vi "log analysis_gps.vi"() -> ()   [LabVIEW 2019] (continued)
\t269.436139\t81.532625\t9.289600\t-0.460581\t-2.044566\t150.612884\t0.332000\t-0.041000\n\t\n15:34:24.6\tlog_raw\tgps_raw\t\tsystem status\tnormal 2 28.000000 0 0\trobot status\t269.315203\t81.615343\t9.281900\t-0.552229\t-2.021285\t150.644029\t0.244000\t0.082000\n\t\n15:34:25.1\tlog_raw\tgps_raw\t\tsystem status\tnormal 2 28.000000 0 0\trobot status\t269.194622\t81.698654\t9.276300\t-0.583893\t-2.101000\t150.710365\t0.325000\t-0.036000\n\t\n15:34:25.6\tlog_raw\tgps_raw\t\tsystem status\tnormal 2 28.000000 0 0\trobot status\t269.074335\t81.783902\t9.271000\t-0.497675\t-2.181605\t150.744108\t0.241000\t0.088000\n\t\n15:34:26.1\tlog_raw\tgps_raw\t\tsystem status\tnormal 2 28.000000 0 0\trobot status\t268.955477\t81.869341\t9.264900\t-0.452583\t-2.247608\t150.742374\t0.270000\t0.036000\n\t\n15:34:26.6\tlog_raw\tgps_raw\t\tsystem status\tnormal 2 28.000000 0 0\trobot status\t268.833115\t81.953814\t9.258000\t-0.503111\t-2.453600\t150.732052\t0.302000\t-0.013000\n\t\n15:34:27.1\tlog_raw\tgps_raw\t\tsystem status\tnormal 2 28.000000 0 0\trobot status\t268.713878\t82.036962\t9.250800\t-0.577483\t-2.510757\t150.712169\t0.246000\t0.079000\n\t\n15:34:27.6\tlog_raw\tgps_raw\t#INSPVAXA,USB3,0,47.0,FINESTEERING,2107,282885.600,02008000,471d,15824;INS_ALIGNMENT_COMPLETE,INS_RTKFIXED,37.37087024505,126.72386724376,9.2438,22.3000,0.1935,-0.2367,-0.0200,-0.555619573,-2.649892401,299.303581082,0.4421,0.2945,0.5549,0.1137,0.0925,0.0774,0.0981,0.1030,4.8706,0f000001,0*97a1aad7\n\tsystem status\tnormal 2 28.000000 0 0\trobot status\t268.581876\t82.129677\t9.243800\t-0.555620\t-2.649892\t150.696419\t0.296000\t0.008000\n\t\n15:34:28.1\tlog_raw\tgps_raw\t\tsystem status\tnormal 2 28.000000 0 0\trobot status\t268.476510\t82.206619\t9.237300\t-0.368024\t-2.541357\t150.675329\t0.256000\t0.056000\n\t\n15:34:28.6\tlog_raw\tgps_raw\t\tsystem status\tnormal 2 28.000000 0 0\trobot status\t268.358117\t82.289532\t9.231700\t-0.318834\t-2.532121\t150.690435\t0.300000\t0.005000\n\t\n15:34:29.1\tlog_raw\tgps_raw\t\tsystem status\tnormal 2 28.000000 0 0\trobot status\t268.240486\t82.371274\t9.225600\t-0.444676\t-2.457903\t150.683698\t0.361000\t-0.089000\n\t\n15:34:29.6\tlog_raw\tgps_raw\t\tsystem status\tnormal 2 28.000000 0 0\trobot status\t268.120488\t82.453127\t9.219200\t-0.577303\t-2.448788\t150.642594\t0.252000\t0.059000\n\t\n15:34:30.1\tlog_raw\tgps_raw\t#INSPVAXA,USB3,0,44.0,FINESTEERING,2107,282888.100,02000000,471d,15824;INS_ALIGNMENT_COMPLETE,INS_RTKFIXED,37.37087398802,126.72386055207,9.2130,22.3000,0.1784,-0.2231,-0.0172,-0.474670007,-2.406033288,299.373176614,0.4412,0.2944,0.5546,0.1136,0.0925,0.0773,0.0980,0.1030,4.8749,0f000001,0*64b8e8ef\n\tsystem status\tnormal 2 28.000000 0 0\trobot status\t267.989137\t82.545108\t9.213000\t-0.474670\t-2.406033\t150.626823\t0.268000\t0.034000\n\t\n15:34:30.6\tlog_raw\tgps_raw\t\tsystem status\tnormal 2 28.000000 0 0\trobot status\t267.880467\t82.621276\t9.207200\t-0.438602\t-2.378533\t150.618241\t0.244000\t0.081000\n\t\n15:34:31.1\tlog_raw\tgps_raw\t\tsystem status\tnormal 2 28.000000 0 0\trobot status\t267.761451\t82.706078\t9.200700\t-0.346891\t-2.412332\t150.574151\t0.282000\t0.019000\n\t\n15:34:31.6\tlog_raw\tgps_raw\t\tsystem status\tnormal 2 28.000000 0 0\trobot status\t267.643575\t82.787980\t9.195000\t-0.379001\t-2.289734\t150.506519\t0.353000\t-0.088000\n\t\n15:34:32.1\tlog_raw\tgps_raw\t\tsystem status\tnormal 2 28.000000 0 0\trobot status\t267.524465\t82.871251\t9.188700\t-0.470678\t-2.248727\t150.509531\t0.253000\t0.060000\n\t\n15:34:32.6\tlog_raw\tgps_raw\t\tsystem status\tnormal 2 28.000000 0 0\trobot status\t267.407071\t82.952609\t9.183600\t-0.561567\t-2.263237\t150.489005\t0.287000\t0.025000\n\t\n15:34:33.1\tlog_raw\tgps_raw\t\tsystem status\tnormal 2 28.000000 0 0\trobot status\t267.291089\t83.035299\t9.177300\t-0.538205\t-2.174307\t150.443336\t0.289000\t0.018000\n\t\n15:34:33.6\tlog_raw\tgps_raw\t\tsystem status\tnormal 2 28.000000 0 0\trobot status\t267.174248\t83.118918\t9.171300\t-0.308620\t-2.273326\t150.485622\t0.327000\t-0.053000\n\t\n15:34:34.1\tlog_raw\tgps_raw\t\tsystem status\tnormal 2 28.000000 0 0\trobot status\t267.055065\t83.203999\t9.166400\t-0.214815\t-2.374419\t150.446306\t0.363000\t-0.110000\n\t\n15:34:34.6\tlog_raw\tgps_raw\t\tsystem status\tnormal 2 28.000000 0 0\trobot status\t266.938684\t83.285845\t9.161300\t-0.295524\t-2.437327\t150.392182\t0.278000\t0.033000\n\t\n15:34:35.1\tlog_raw\tgps_raw\t\tsystem status\tnormal 2 28.000000 0 0\trobot status\t266.824358\t83.368135\t9.157000\t-0.276386\t-2.328868\t150.443706\t0.279000\t0.029000\n\t\n15:34:35.6\tlog_raw\tgps_raw\t\tsystem status\tnormal 2 28.000000 0 0\trobot status\t266.706166\t83.452437\t9.153400\t-0.267022\t-2.347712\t150.469778\t0.323000\t-0.044000\n\t\n15:34:36.1\tlog_raw\tgps_raw\t\tsystem status\tnormal 2 28.000000 0 0\trobot status\t266.589120\t83.537244\t9.150100\t-0.269755\t-2.340895\t150.478741\t0.285000\t0.026000\n\t\n15:34:36.6\tlog_raw\tgps_raw\t\tsystem status\tnormal 2 28.000000 0 0\trobot status\t266.475594\t83.619238\t9.146900\t-0.192257\t-2.213213\t150.498544\t0.384000\t-0.112000\n\t\n15:34:37.1\tlog_raw\tgps_raw\t#INSPVAXA,USB3,0,48.5,FINESTEERING,2107,282895.100,02000000,471d,15824;INS_ALIGNMENT_COMPLETE,INS_RTKFIXED,37.37088448799,126.72384205034,9.1438,22.3000,0.1933,-0.2424,-0.0028,-0.201390353,-2.093342605,299.449772344,0.4447,0.2945,0.5555,0.1140,0.0925,0.0774,0.0980,0.1030,4.8838,0f000001,0*927e2c09\n\tsystem status\tnormal 2 27.900000 0 0\trobot status\t266.350284\t83.710495\t9.143800\t-0.201390\t-2.093343\t150.550228\t0.262000\t0.069000\n\t\n15:34:37.6\tlog_raw\tgps_raw\t#INSPVAXA,USB3,0,48.5,FINESTEERING,2107,282895.600,02000000,471d,15824;INS_ALIGNMENT_COMPLETE,INS_RTKFIXED,37.37088525085,126.72384071933,9.1382,22.3000,0.1891,-0.2249,-0.0147,-0.298436977,-2.149365506,299.431607145,0.4447,0.2945,0.5555,0.1140,0.0925,0.0774,0.0980,0.1030,4.8838,0f000001,0*8cb89ae5\n\tsystem status\tnormal 2 27.900000 0 0\trobot status\t266.232386\t83.795165\t9.138200\t-0.298437\t-2.149366\t150.568393\t0.281000\t0.032000\n\t\n15:34:38.1\tlog_raw\tgps_raw\t#INSPVAXA,USB3,0,50.0,FINESTEERING,2107,282896.100,02000000,471d,15824;INS_ALIGNMENT_COMPLETE,INS_RTKFIXED,37.37088602098,126.72383942643,9.1321,22.3000,0.1872,-0.2208,-0.0098,-0.216671820,-2.100330729,299.377504290,0.4449,0.2945,0.5555,0.1140,0.0925,0.0774,0.0980,0.1030,4.8845,0f000001,0*ef0b4927\n\tsystem status\tnormal 2 28.000000 0 0\trobot status\t266.117863\t83.880641\t9.132100\t-0.216672\t-2.100331\t150.622496\t0.265000\t0.063000\n\t\n15:34:38.6\tlog_raw\tgps_raw\t#INSPVAXA,USB3,0,50.0,FINESTEERING,2107,282896.600,02000000,471d,15824;INS_ALIGNMENT_COMPLETE,INS_RTKFIXED,37.37088675072,126.72383814980,9.1274,22.3000,0.1877,-0.2084,-0.0156,-0.228208842,-2.023017787,299.331781816,0.4449,0.2945,0.5555,0.1140,0.0925,0.0774,0.0980,0.1030,4.8845,0f000001,0*c594017f\n\tsystem status\tnormal 2 28.000000 0 0\trobot status\t266.004781\t83.961635\t9.127400\t-0.228209\t-2.023018\t150.668218\t0.285000\t0.024000\n\t\n15:34:39.1\tlog_raw\tgps_raw\t#INSPVAXA,USB3,0,50.5,FINESTEERING,2107,282897.100,02000000,471d,15824;INS_ALIGNMENT_COMPLETE,INS_RTKFIXED,37.37088750252,126.72383685308,9.1243,22.3000,0.1876,-0.2107,-0.0114,-0.201079382,-2.183646945,299.196189709,0.4447,0.2943,0.5554,0.1139,0.0925,0.0774,0.0980,0.1030,4.8850,0f000001,0*259ceb0e\n\tsystem status\tnormal 2 28.000000 0 0\trobot status\t265.889920\t84.045076\t9.124300\t-0.201079\t-2.183647\t150.803810\t0.274000\t0.040000\n\t\n15:34:39.6\tlog_raw\tgps_raw\t#INSPVAXA,USB3,0,50.5,FINESTEERING,2107,282897.600,02000000,471d,15824;INS_ALIGNMENT_COMPLETE,INS_RTKFIXED,37.37088825874,126.72383552871,9.1219,22.3000,0.1981,-0.2184,-0.0197,-0.162513691,-2.197478943,299.137776460,0.4447,0.2943,0.5554,0.1139,0.0925,0.0774,0.0980,0.1030,4.8850,0f000001,0*0c5abc39\n\tsystem status\tnormal 2 28.000000 0 0\trobot status\t265.772609\t84.129009\t9.121900\t-0.162514\t-2.197479\t150.862224\t0.353000\t-0.063000\n\t\n15:34:40.1\tlog_raw\tgps_raw\t#INSPVAXA,USB3,0,49.5,FINESTEERING,2107,282898.100,02000000,471d,15824;INS_ALIGNMENT_COMPLETE,INS_RTKFIXED,37.37088900648,126.72383424276,9.1196,22.3000,0.2094,-0.2215,-0.0185,-0.097507181,-2.148657540,298.990101476,0.4444,0.2942,0.5550,0.1138,0.0925,0.0774,0.0981,0.1030,4.8854,0f000001,0*b8bcb2e5\n\tsystem status\tnormal 2 27.900000 0 0\trobot status\t265.658702\t84.212000\t9.119600\t-0.097507\t-2.148658\t151.009899\t0.277000\t0.042000\n\t\n15:34:40.6\tlog_raw\tgps_raw\t\tsystem status\tnormal 2 27.900000 0 0\trobot status\t265.555116\t84.286064\t9.116100\t-0.033377\t-2.065894\t151.068145\t0.247000\t0.094000\n\t\n15:34:41.1\tlog_raw\tgps_raw\t\tsystem status\tnormal 2 28.000000 0 0\trobot status\t265.437719\t84.369636\t9.111700\t-0.021479\t-2.037968\t151.178463\t0.448000\t-0.221000\n\t\n15:34:41.6\tlog_raw\tgps_raw\t\tsystem status\tnormal 2 27.900000 0 0\trobot status\t265.321293\t84.451017\t9.109300\t0.038913\t-2.028452\t151.267255\t0.273000\t0.055000\n\t\n15:34:42.1\tlog_raw\tgps_raw\t\tsystem status\tnormal 2 27.900000 0 0\trobot status\t265.205758\t84.531606\t9.106900\t-0.067838\t-1.982593\t151.367214\t0.234000\t0.111000\n\t\n15:34:42.6\tlog_raw\tgps_raw\t\tsystem status\tnormal 2 27.900000 0 0\trobot status\t265.087725\t84.613924\t9.104700\t0.030629\t-2.066884\t151.494607\t0.249000\t0.072000\n\t\n15:34:43.1\tlog_raw\tgps_raw\t#INSPVAXA,USB3,0,44.5,FINESTEERING,2107,282901.100,02000000,471d,15824;INS_ALIGNMENT_COMPLETE,INS_RTKFIXED,37.37089345276,126.72382632257,9.1013,22.3000,0.2073,-0.2174,-0.0049,0.127947696,-2.049748095,298.428012229,0.4429,0.2942,0.5542,0.1136,0.0924,0.0773,0.0981,0.1029,4.8869,0f000001,0*2739f994\n\tsystem status\tnormal 2 27.900000 0 0\trobot status\t264.957144\t84.705491\t9.101300\t0.127948\t-2.049748\t151.571988\t0.351000\t-0.065000\n\t\n15:34:43.6\tlog_raw\tgps_raw\t#INSPVAXA,USB3,0,44.5,FINESTEERING,2107,282901.600,02000000,471d,15824;INS_ALIGNMENT_COMPLETE,INS_RTKFIXED,37.37089417130,126.72382498099,9.0979,22.3000,0.2123,-0.2139,-0.0112,0.110382768,-2.113702114,298.389030042,0.4429,0.2942,0.5542,0.1136,0.0924,0.0773,0.0981,0.1029,4.8869,0f000001,0*7ea02078\n\tsystem status\tnormal 2 27.900000 0 0\trobot status\t264.838309\t84.785242\t9.097900\t0.110383\t-2.113702\t151.610970\t0.439000\t-0.195000\n\t\n15:34:44.1\tlog_raw\tgps_raw\t#INSPVAXA,USB3,0,47.5,FINESTEERING,2107,282902.100,02000000,471d,15824;INS_ALIGNMENT_COMPLETE,INS_RTKFIXED,37.37089489898,126.72382363217,9.0942,22.3000,0.2058,-0.2206,-0.0113,0.048071178,-2.299077036,298.376589904,0.4428,0.2943,0.5540,0.1136,0.0924,0.0773,0.0981,0.1029,4.8877,0f000001,0*27878755\n\tsystem status\tnormal 2 28.000000 0 0\trobot status\t264.718833\t84.866007\t9.094200\t0.048071\t-2.299077\t151.623410\t0.221000\t0.136000\n\t\n15:34:44.6\tlog_raw\tgps_raw\t#INSPVAXA,USB3,0,47.5,FINESTEERING,2107,282902.600,02000000,471d,15824;INS_ALIGNMENT_COMPLETE,INS_RTKFIXED,37.37089561933,126.72382228336,9.0897,22.3000,0.2051,-0.2120,-0.0118,0.043026481,-2.382631281,298.375025440,0.4428,0.2943,0.5540,0.1136,0.0924,0.0773,0.0981,0.1029,4.8877,0f000001,0*7b155814\n\tsystem status\tnormal 2 28.000000 0 0\trobot status\t264.599358\t84.945958\t9.089700\t0.043026\t-2.382631\t151.624975\t0.344000\t-0.069000\n\t\n15:34:45.1\tlog_raw\tgps_raw\t#INSPVAXA,USB3,0,50.5,FINESTEERING,2107,282903.100,02000000,471d,15824;INS_ALIGNMENT_COMPLETE,INS_RTKFIXED,37.37089633791,126.72382096695,9.0851,22.3000,0.2033,-0.2166,-0.0158,0.077766570,-2.447937912,298.353889057,0.4425,0.2944,0.5540,0.1136,0.0924,0.0773,0.0981,0.1029,4.8888,0f000001,0*d3856956\n\tsystem status\tnormal 2 28.000000 0 0\trobot status\t264.482752\t85.025713\t9.085100\t0.077767\t-2.447938\t151.646111\t0.409000\t-0.173000\n\t\n15:34:45.6\tlog_raw\tgps_raw\t#INSPVAXA,USB3,0,50.5,FINESTEERING,2107,282903.600,02000000,471d,15824;INS_ALIGNMENT_COMPLETE,INS_RTKFIXED,37.37089705589,126.72381965369,9.0797,22.3000,0.2030,-0.2155,-0.0169,0.162662561,-2.490332346,298.323964728,0.4425,0.2944,0.5540,0.1136,0.0924,0.0773,0.0981,0.1029,4.8888,0f000001,0*903bf558\n\tsystem status\tnormal 2 28.000000 0 0\trobot status\t264.366426\t85.105402\t9.079700\t0.162663\t-2.490332\t151.676035\t0.328000\t-0.052000\n\t\n15:34:46.1\tlog_raw\tgps_raw\t#INSPVAXA,USB3,0,48.5,FINESTEERING,2107,282904.100,02000000,471d,15824;INS_ALIGNMENT_COMPLETE,INS_RTKFIXED,37.37089779647,126.72381832272,9.0739,22.3000,0.1899,-0.2136,-0.0154,0.294805164,-2.652846307,298.299564354,0.4429,0.2945,0.5544,0.1137,0.0925,0.0774,0.0981,0.1030,4.8900,0f000001,0*1aba8cff\n\tsystem status\tnormal 2 28.000000 0 0\trobot status\t264.248531\t85.187598\t9.073900\t0.294805\t-2.652846\t151.700436\t0.281000\t0.007000\n\t\n15:34:46.6\tlog_raw\tgps_raw\t\tsystem status\tnormal 2 28.000000 0 0\trobot status\t264.139827\t85.260598\t9.068300\t0.313257\t-2.570583\t151.646867\t0.257000\t0.059000\n\t\n15:34:47.1\tlog_raw\tgps_raw\t#INSPVAXA,USB3,0,42.5,FINESTEERING,2107,282905.100,02000000,471d,15824;INS_ALIGNMENT_COMPLETE,INS_RTKFIXED,37.37089924281,126.72381565825,9.0621,22.3000,0.2032,-0.2264,-0.0151,0.296199790,-2.500120429,298.405278935,0.4415,0.2943,0.5538,0.1135,0.0924,0.0773,0.0981,0.1029,4.8913,0f000001,0*c27d96a4\n\tsystem status\tnormal 2 28.000000 0 0\trobot status\t264.012516\t85.348127\t9.062100\t0.296200\t-2.500120\t151.594721\t0.253000\t0.070000\n\t\n15:34:47.6\tlog_raw\tgps_raw\t#INSPVAXA,USB3,0,42.5,FINESTEERING,2107,282905.600,02000000,471d,15824;INS_ALIGNMENT_COMPLETE,INS_RTKFIXED,37.37089993990,126.72381433650,9.0561,22.3000,0.1965,-0.2206,-0.0194,0.175024687,-2.429152117,298.413626254,0.4415,0.2943,0.5538,0.1135,0.0924,0.0773,0.0981,0.1029,4.8913,0f000001,0*60204f40\n\tsystem status\tnormal 2 28.000000 0 0\trobot status\t263.895438\t85.425497\t9.056100\t0.175025\t-2.429152\t151.586374\t0.255000\t0.060000\n\t\n15:34:48.1\tlog_raw\tgps_raw\t#INSPVAXA,USB3,0,50.0,FINESTEERING,2107,282906.100,02000000,471d,15824;INS_ALIGNMENT_COMPLETE,INS_RTKFIXED,37.37090067392,126.72381297631,9.0488,22.3000,0.1869,-0.2231,-0.0278,0.198226586,-2.470510374,298.476445158,0.4408,0.2943,0.5536,0.1134,0.0924,0.0773,0.0981,0.1029,4.8926,0f000001,0*c8d31ab7\n\tsystem status\tnormal 2 28.000000 0 0\trobot status\t263.774954\t85.506966\t9.048800\t0.198227\t-2.470510\t151.523555\t0.243000\t0.074000\n\t\n15:34:48.6\tlog_raw\tgps_raw\t#INSPVAXA,USB3,0,50.0,FINESTEERING,2107,282906.600,02000000,471d,15824;INS_ALIGNMENT_COMPLETE,INS_RTKFIXED,37.37090140156,126.72381162044,9.0410,22.3000,0.1900,-0.2268,-0.0250,0.233406583,-2.464396388,298.527307451,0.4408,0.2943,0.5536,0.1134,0.0924,0.0773,0.0981,0.1029,4.8926,0f000001,0*6dbb954e\n\tsystem status\tnormal 2 28.000000 0 0\trobot status\t263.654854\t85.587727\t9.041000\t0.233407\t-2.464396\t151.472693\t0.249000\t0.074000\n\t\n15:34:49.1\tlog_raw\tgps_raw\t#INSPVAXA,USB3,0,47.5,FINESTEERING,2107,282907.100,02000000,471d,15824;INS_ALIGNMENT_COMPLETE,INS_RTKFIXED,37.37090211288,126.72381031698,9.0345,22.3000,0.1914,-0.2193,-0.0163,0.234265658,-2.429917565,298.557656131,0.4407,0.2944,0.5534,0.1135,0.0925,0.0773,0.0981,0.1029,4.8940,0f000001,0*98d66c71\n\tsystem status\tnormal 2 28.000000 0 0\trobot status\t263.539395\t85.666676\t9.034500\t0.234266\t-2.429918\t151.442344\t0.281000\t0.006000\n\t\n15:34:49.6\tlog_raw\tgps_raw\t#INSPVAXA,USB3,0,47.5,FINESTEERING,2107,282907.600,02000000,471d,15824;INS_ALIGNMENT_COMPLETE,INS_RTKFIXED,37.37090284953,126.72380892748,9.0281,22.3000,0.1780,-0.2041,-0.0150,0.112459051,-2.561733911,298.657756217,0.4407,0.2944,0.5534,0.1135,0.0925,0.0773,0.0981,0.1029,4.8940,0f000001,0*46e93b24\n\tsystem status\tnormal 2 28.000000 0 0\trobot status\t263.416316\t85.748437\t9.028100\t0.112459\t-2.561734\t151.342244\t0.249000\t0.069000\n\t\n15:34:50.1\tlog_raw\tgps_raw\t#INSPVAXA,USB3,0,47.5,FINESTEERING,2107,282908.100,02000000,471d,15824;INS_ALIGNMENT_COMPLETE,INS_RTKFIXED,37.37090357557,126.72380757332,9.0217,22.3000,0.2057,-0.2321,-0.0149,0.061524953,-2.489801509,298.773706778,0.4409,0.2944,0.5534,0.1134,0.0925,0.0773,0.0981,0.1029,4.8951,0f000001,0*737dd3e1\n\tsystem status\tnormal 2 28.000000 0 0\trobot status\t263.296366\t85.829020\t9.021700\t0.061525\t-2.489802\t151.226293\t0.296000\t0.003000\n\t\n15:34:50.6\tlog_raw\tgps_raw\t#INSPVAXA,USB3,0,42.5,FINESTEERING,2107,282908.600,02000000,471d,15824;INS_ALIGNMENT_COMPLETE,INS_RTKFIXED,37.37090428415,126.72380622581,9.0150,22.3000,0.1993,-0.2229,-0.0194,0.018544103,-2.459857959,298.845685977,0.4409,0.2944,0.5534,0.1134,0.0925,0.0773,0.0981,0.1029,4.8951,0f000001,0*f932705e\n\tsystem status\tnormal 2 28.000000 0 0\trobot status\t263.177006\t85.907665\t9.015000\t0.018544\t-2.459858\t151.154314\t0.276000\t0.024000\n\t\n15:34:51.1\tlog_raw\tgps_raw\t#INSPVAXA,USB3,0,45.5,FINESTEERING,2107,282909.100,02000000,471d,15824;INS_ALIGNMENT_COMPLETE,INS_RTKFIXED,37.37090502254,126.72380483216,9.0074,22.3000,0.1877,-0.2104,-0.0206,-0.090329657,-2.475798603,298.940458629,0.4409,0.2946,0.5535,0.1135,0.0926,0.0773,0.0981,0.1029,4.8962,0f000001,0*a1f88c2d\n\tsystem status\tnormal 2 28.000000 0 0\trobot status\t263.053559\t85.989619\t9.007400\t-0.090330\t-2.475799\t151.059541\t0.249000\t0.062000\n\t\n15:34:51.6\tlog_raw\tgps_raw\t#INSPVAXA,USB3,0,45.5,FINESTEERING,2107,282909.600,02000000,471d,15824;INS_ALIGNMENT_COMPLETE,INS_RTKFIXED,37.37090578020,126.72380341402,9.0005,22.3000,0.2042,-0.2452,-0.0267,-0.096054371,-2.657817318,299.053399996,0.4409,0.2946,0.5535,0.1135,0.0926,0.0773,0.0981,0.1029,4.8962,0f000001,0*97d4220e\n\tsystem status\tnormal 2 28.000000 0 0\trobot status\t262.927942\t86.073711\t9.000500\t-0.096054\t-2.657817\t150.946600\t0.311000\t-0.024000\n\t\n15:34:52.1\tlog_raw\tgps_raw\t#INSPVAXA,USB3,0,44.5,FINESTEERING,2107,282910.100,02000000,471d,15824;INS_ALIGNMENT_COMPLETE,INS_RTKFIXED,37.37090649384,126.72380213526,8.9945,22.3000,0.1796,-0.2032,-0.0123,-0.081156055,-2.596786574,299.082136119,0.4412,0.2947,0.5535,0.1135,0.0926,0.0773,0.0981,0.1029,4.8970,0f000001,0*70e9c9df\n\tsystem status\tnormal 2 28.000000 0 0\trobot status\t262.814672\t86.152918\t8.994500\t-0.081156\t-2.596787\t150.917864\t0.270000\t0.031000\n\t\n15:34:52.6\tlog_raw\tgps_raw\t#INSPVAXA,USB3,0,44.5,FINESTEERING,2107,282910.600,02000000,471d,15824;INS_ALIGNMENT_COMPLETE,INS_RTKFIXED,37.37090728426,126.72380074897,8.9873,22.3000,0.2078,-0.2346,-0.0218,0.045801771,-2.674891598,299.142927174,0.4412,0.2947,0.5535,0.1135,0.0926,0.0773,0.0981,0.1029,4.8970,0f000001,0*500925c1\n\tsystem status\tnormal 2 28.000000 0 0\trobot status\t262.691877\t86.240646\t8.987300\t0.045802\t-2.674892\t150.857073\t0.306000\t-0.009000\n\t\n15:34:53.1\tlog_raw\tgps_raw\t#INSPVAXA,USB3,0,45.5,FINESTEERING,2107,282911.100,02000000,471d,15824;INS_ALIGNMENT_COMPLETE,INS_RTKFIXED,37.37090803309,126.72379945819,8.9800,22.3000,0.1796,-0.1956,-0.0242,0.023894528,-2.705451433,299.250076985,0.4415,0.2948,0.5535,0.1135,0.0925,0.0773,0.0981,0.1029,4.8973,0f000001,0*fcb889be\n\tsystem status\tnormal 2 28.000000 0 0\trobot status\t262.577542\t86.323758\t8.980000\t0.023895\t-2.705451\t150.749923\t0.328000\t-0.060000\n\t\n15:34:53.6\tlog_raw\tgps_raw\t#INSPVAXA,USB3,0,45.5,FINESTEERING,2107,282911.600,02000000,471d,15824;INS_ALIGNMENT_COMPLETE,INS_RTKFIXED,37.37090882517,126.72379803977,8.9729,22.3000,0.1992,-0.2347,-0.0122,-0.052701655,-2.537774269,299.314444801,0.4415,0.2948,0.5535,0.1135,0.0925,0.0773,0.0981,0.1029,4.8973,0f000001,0*f806d9f3\n\tsystem status\tnormal 2 28.000000 0 0\trobot status\t262.451900\t86.411671\t8.972900\t-0.052702\t-2.537774\t150.685555\t0.302000\t-0.007000\n\t\n15:34:54.1\tlog_raw\tgps_raw\t#INSPVAXA,USB3,0,49.0,FINESTEERING,2107,282912.100,02000000,471d,15824;INS_ALIGNMENT_COMPLETE,INS_RTKFIXED,37.37090954144,126.72379680635,8.9662,22.3000,0.2005,-0.2326,-0.0241,-0.125797305,-2.436851943,299.381095140,0.4412,0.2948,0.5534,0.1134,0.0926,0.0773,0.0980,0.1029,4.8978,0f000001,0*e5b9f40a\n\tsystem status\tnormal 2 28.000000 0 0\trobot status\t262.342646\t86.491169\t8.966200\t-0.125797\t-2.436852\t150.618905\t0.288000\t0.006000\n\t\n15:34:54.6\tlog_raw\tgps_raw\t#INSPVAXA,USB3,0,49.0,FINESTEERING,2107,282912.600,02000000,471d,15824;INS_ALIGNMENT_COMPLETE,INS_RTKFIXED,37.37091031837,126.72379541279,8.9597,22.3000,0.1852,-0.2068,-0.0204,-0.071142448,-2.486574172,299.492569727,0.4412,0.2948,0.5534,0.1134,0.0926,0.0773,0.0980,0.1029,4.8978,0f000001,0*cac4ba0d\n\tsystem status\tnormal 2 28.000000 0 0\trobot status\t262.219207\t86.577401\t8.959700\t-0.071142\t-2.486574\t150.507430\t0.229000\t0.086000\n\t\n15:34:55.1\tlog_raw\tgps_raw\t#INSPVAXA,USB3,0,49.5,FINESTEERING,2107,282913.100,02000000,471d,15824;INS_ALIGNMENT_COMPLETE,INS_RTKFIXED,37.37091108524,126.72379405931,8.9519,22.3000,0.1888,-0.2272,-0.0247,-0.028725670,-2.337365397,299.552597059,0.4407,0.2948,0.5532,0.1133,0.0925,0.0773,0.0980,0.1028,4.8983,0f000001,0*e96bcee1\n\tsystem status\tnormal 2 28.000000 0 0\trobot status\t262.099318\t86.662515\t8.951900\t-0.028726\t-2.337365\t150.447403\t0.289000\t0.015000\n\t\n15:34:55.6\tlog_raw\tgps_raw\t#INSPVAXA,USB3,0,49.5,FINESTEERING,2107,282913.600,02000000,471d,15824;INS_ALIGNMENT_COMPLETE,INS_RTKFIXED,37.37091181929,126.72379275953,8.9460,22.3000,0.2010,-0.2341,-0.0266,0.089811982,-2.060196464,299.576677056,0.4407,0.2948,0.5532,0.1133,0.0925,0.0773,0.0980,0.1028,4.8983,0f000001,0*1320fd5f\n\tsystem status\tnormal 2 28.000000 0 0\trobot status\t261.984185\t86.743987\t8.946000\t0.089812\t-2.060196\t150.423323\t0.349000\t-0.076000\n\t\n15:34:56.1\tlog_raw\tgps_raw\t#DUALANTENNAHEADINGA,USB3,0,49.5,FINESTEERING,2107,282914.100,02000000,d426,15824;INSUFFICIENT_OBS,NONE,-1.000000000,0.000000000,0.000000000,0.0,0.000000000,0.000000000,\"631T\",13,2,2,2,04,00,20,00*7d7777a8\n\tsystem status\tnormal 2 28.000000 0 0\trobot status\t261.864200\t86.827130\t8.939200\t-0.070666\t-2.033883\t150.415109\t0.253000\t0.066000\n\t\n15:34:56.6\tlog_raw\tgps_raw\t#INSPVAXA,USB3,0,52.5,FINESTEERING,2107,282914.600,02000000,471d,15824;INS_ALIGNMENT_COMPLETE,INS_RTKFIXED,37.37091330951,126.72379003668,8.9325,22.3000,0.2030,-0.2221,-0.0237,-0.171357010,-2.043364935,299.558430803,0.4402,0.2946,0.5530,0.1134,0.0925,0.0773,0.0980,0.1028,4.8991,0f000001,0*e9175f83\n\tsystem status\tnormal 2 28.000000 0 0\trobot status\t261.743000\t86.909386\t8.932500\t-0.171357\t-2.043365\t150.441569\t0.258000\t0.063000\n\t\n15:34:57.1\tlog_raw\tgps_raw\t#INSPVAXA,USB3,0,50.0,FINESTEERING,2107,282915.100,02000000,471d,15824;INS_ALIGNMENT_COMPLETE,INS_RTKFIXED,37.37091408421,126.72378863973,8.9262,22.3000,0.1969,-0.2337,-0.0140,-0.095383380,-2.265013961,299.603418262,0.4401,0.2946,0.5529,0.1132,0.0924,0.0773,0.0980,0.1028,4.8997,0f000001,0*6f852fd6\n\tsystem status\tnormal 2 28.000000 0 0\trobot status\t261.619260\t86.995370\t8.926200\t-0.095383\t-2.265014\t150.396582\t0.255000\t0.060000\n\t\n15:34:57.6\tlog_raw\tgps_raw\t#DUALANTENNAHEADINGA,USB3,0,50.0,FINESTEERING,2107,282915.600,02000000,d426,15824;INSUFFICIENT_OBS,NONE,-1.000000000,0.000000000,0.000000000,0.0,0.000000000,0.000000000,\"631T\",17,2,2,2,04,00,20,00*414acee8\n\tsystem status\tnormal 2 28.000000 0 0\trobot status\t261.500918\t87.077460\t8.921500\t-0.059833\t-2.292781\t150.397040\t0.297000\t0.006000\n\t\n15:34:58.1\tlog_raw\tgps_raw\t#DUALANTENNAHEADINGA,USB3,0,48.5,FINESTEERING,2107,282916.100,02000000,d426,15824;INSUFFICIENT_OBS,NONE,-1.000000000,0.000000000,0.000000000,0.0,0.000000000,0.000000000,\"631T\",16,2,2,2,04,00,20,00*fc092504\n\tsystem status\tnormal 2 28.000000 0 0\trobot status\t261.379338\t87.160459\t8.916300\t-0.201226\t-2.330521\t150.547227\t0.285000\t0.028000\n\t\n15:34:58.6\tlog_raw\tgps_raw\t#INSPVAXA,USB3,0,48.5,FINESTEERING,2107,282916.600,02000000,471d,15824;INS_ALIGNMENT_COMPLETE,INS_RTKFIXED,37.37091631932,126.72378455605,8.9095,22.3000,0.1948,-0.2448,-0.0204,-0.186363479,-2.427120198,299.446159990,0.4395,0.2945,0.5529,0.1132,0.0924,0.0773,0.0979,0.1028,4.9009,0f000001,0*c1989546\n\tsystem status\tnormal 2 28.000000 0 0\trobot status\t261.257534\t87.243444\t8.909500\t-0.186363\t-2.427120\t150.553840\t0.289000\t0.009000\n\t\n15:34:59.1\tlog_raw\tgps_raw\t#INSPVAXA,USB3,0,49.0,FINESTEERING,2107,282917.100,02000000,471d,15824;INS_ALIGNMENT_COMPLETE,INS_RTKFIXED,37.37091707280,126.72378318034,8.9014,22.3000,0.1962,-0.2403,-0.0192,-0.090528151,-2.520576171,299.333268916,0.4392,0.2943,0.5527,0.1132,0.0925,0.0773,0.0979,0.1028,4.9023,0f000001,0*ed058076\n\tsystem status\tnormal 2 27.900000 0 0\trobot status\t261.135676\t87.327072\t8.901400\t-0.090528\t-2.520576\t150.666731\t0.298000\t-0.006000\n\t\n15:34:59.6\tlog_raw\tgps_raw\t#INSPVAXA,USB3,0,49.0,FINESTEERING,2107,282917.600,02000000,471d,15824;INS_ALIGNMENT_COMPLETE,INS_RTKFIXED,37.37091780195,126.72378182721,8.8930,22.3000,0.1904,-0.2448,-0.0126,-0.105477255,-2.530837408,299.214922397,0.4392,0.2943,0.5527,0.1132,0.0925,0.0773,0.0979,0.1028,4.9023,0f000001,0*48e5530c\n\tsystem status\tnormal 2 28.000000 0 0\trobot status\t261.015818\t87.408000\t8.893000\t-0.105477\t-2.530837\t150.785078\t0.219000\t0.123000\n\t\n15:35:00.1\tlog_raw\tgps_raw\t#INSPVAXA,USB3,0,49.5,FINESTEERING,2107,282918.100,02000000,471d,15824;INS_ALIGNMENT_COMPLETE,INS_RTKFIXED,37.37091853728,126.72378045121,8.8866,22.3000,0.1905,-0.2390,-0.0217,-0.320620124,-2.745936216,299.166142272,0.4393,0.2944,0.5528,0.1133,0.0925,0.0773,0.0979,0.1028,4.9038,0f000001,0*f3e51291\n\tsystem status\tnormal 2 28.000000 0 0\trobot status\t260.893934\t87.489614\t8.886600\t-0.320620\t-2.745936\t150.833858\t0.298000\t0.003000\n\t\n15:35:00.6\tlog_raw\tgps_raw\t#INSPVAXA,USB3,0,49.5,FINESTEERING,2107,282918.600,02000000,471d,15824;INS_ALIGNMENT_COMPLETE,INS_RTKFIXED,37.37091927039,126.72377907949,8.8817,22.3000,0.1978,-0.2407,-0.0282,-0.339255571,-2.778752767,299.132032456,0.4393,0.2944,0.5528,0.1133,0.0925,0.0773,0.0979,0.1028,4.9038,0f000001,0*ae621dff\n\tsystem status\tnormal 2 28.000000 0 0\trobot status\t260.772430\t87.570982\t8.881700\t-0.339256\t-2.778753\t150.867968\t0.431000\t-0.195000\n\t\n15:35:01.1\tlog_raw\tgps_raw\t#INSPVAXA,USB3,0,45.0,FINESTEERING,2107,282919.100,02000000,471d,15824;INS_ALIGNMENT_COMPLETE,INS_RTKFIXED,37.37092001431,126.72377771681,8.8758,22.3000,0.1914,-0.2350,-0.0323,-0.346867597,-2.754638155,299.109102683,0.4397,0.2944,0.5532,0.1134,0.0925,0.0773,0.0979,0.1029,4.9053,0f000001,0*63db1984\n\tsystem status\tnormal 2 27.900000 0 0\trobot status\t260.651726\t87.653550\t8.875800\t-0.346868\t-2.754638\t150.890897\t0.350000\t-0.072000\n\t\n15:35:01.6\tlog_raw\tgps_raw\t#INSPVAXA,USB3,0,45.0,FINESTEERING,2107,282919.600,02000000,471d,15824;INS_ALIGNMENT_COMPLETE,INS_RTKFIXED,37.37092075682,126.72377638763,8.8692,22.3000,0.1933,-0.2372,-0.0282,-0.392529438,-2.688019024,299.098365705,0.4397,0.2944,0.5532,0.1134,0.0925,0.0773,0.0979,0.1029,4.9053,0f000001,0*15ef86f5\n\tsystem status\tnormal 2 28.000000 0 0\trobot status\t260.533989\t87.735960\t8.869200\t-0.392529\t-2.688019\t150.901634\t0.326000\t-0.035000\n\t\n15:35:02.1\tlog_raw\tgps_raw\t#INSPVAXA,USB3,0,45.0,FINESTEERING,2107,282920.100,02000000,471d,15824;INS_ALIGNMENT_COMPLETE,INS_RTKFIXED,37.37092151983,126.72377503879,8.8627,22.3000,0.1947,-0.2324,-0.0288,-0.374754303,-2.758160229,299.096118379,0.4395,0.2945,0.5534,0.1133,0.0925,0.0773,0.0980,0.1029,4.9066,0f000001,0*6a5bdc77\n\tsystem status\tnormal 2 28.000000 0 0\trobot status\t260.414511\t87.820647\t8.862700\t-0.374754\t-2.758160\t150.903882\t0.418000\t-0.168000\n\t\n15:35:02.6\tlog_raw\tgps_raw\t#INSPVAXA,USB3,0,50.0,FINESTEERING,2107,282920.600,02000000,471d,15824;INS_ALIGNMENT_COMPLETE,INS_RTKFIXED,37.37092225918,126.72377371320,8.8579,22.3000,0.2080,-0.2433,-0.0263,-0.353123452,-2.702710853,299.168531612,0.4395,0.2945,0.5534,0.1133,0.0925,0.0773,0.0980,0.1029,4.9066,0f000001,0*b7196621\n\tsystem status\tnormal 2 28.000000 0 0\trobot status\t260.297092\t87.902707\t8.857900\t-0.353123\t-2.702711\t150.831468\t0.294000\t0.019000\n\t\n15:35:03.1\tlog_raw\tgps_raw\t#DUALANTENNAHEADINGA,USB3,0,50.0,FINESTEERING,2107,282921.100,02000000,d426,15824;INSUFFICIENT_OBS,NONE,-1.000000000,0.000000000,0.000000000,0.0,0.000000000,0.000000000,\"631T\",10,2,2,2,04,00,20,00*711b9acd\n\tsystem status\tnormal 2 28.000000 0 0\trobot status\t260.180847\t87.984238\t8.853900\t-0.343319\t-2.734939\t150.851400\t0.286000\t0.026000\n\t\n15:35:03.6\tlog_raw\tgps_raw\t#INSPVAXA,USB3,0,51.0,FINESTEERING,2107,282921.600,02000000,471d,15824;INS_ALIGNMENT_COMPLETE,INS_RTKFIXED,37.37092372084,126.72377106985,8.8494,22.3000,0.2060,-0.2301,-0.0270,-0.435271636,-2.731976151,299.129546059,0.4391,0.2944,0.5533,0.1133,0.0925,0.0773,0.0980,0.1029,4.9078,0f000001,0*5c44fd03\n\tsystem status\tnormal 2 28.000000 0 0\trobot status\t260.062949\t88.064936\t8.849400\t-0.435272\t-2.731976\t150.870454\t0.376000\t-0.116000\n\t\n15:35:04.1\tlog_raw\tgps_raw\t#DUALANTENNAHEADINGA,USB3,0,51.0,FINESTEERING,2107,282922.100,02000000,d426,15824;INSUFFICIENT_OBS,NONE,-1.000000000,0.000000000,0.000000000,0.0,0.000000000,0.000000000,\"631T\",12,2,2,2,04,00,20,00*d78347f3\n\tsystem status\tnormal 2 28.000000 0 0\trobot status\t259.944761\t88.147198\t8.844200\t-0.331286\t-2.658657\t150.844836\t0.286000\t0.017000\n\t\n15:35:04.6\tlog_raw\tgps_raw\t#INSPVAXA,USB3,0,51.0,FINESTEERING,2107,282922.600,02000000,471d,15824;INS_ALIGNMENT_COMPLETE,INS_RTKFIXED,37.37092515994,126.72376843182,8.8389,22.3000,0.2111,-0.2302,-0.0297,-0.438503525,-2.449777885,299.109289893,0.4389,0.2944,0.5534,0.1132,0.0925,0.0773,0.0980,0.1029,4.9089,0f000001,0*6200cf77\n\tsystem status\tnormal 2 28.000000 0 0\trobot status\t259.829276\t88.224661\t8.838900\t-0.438504\t-2.449778\t150.890710\t0.250000\t0.077000\n\t\n15:35:05.1\tlog_raw\tgps_raw\t#DUALANTENNAHEADINGA,USB3,0,50.0,FINESTEERING,2107,282923.100,02000000,d426,15824;INSUFFICIENT_OBS,NONE,-1.000000000,0.000000000,0.000000000,0.0,0.000000000,0.000000000,\"631T\",13,2,2,2,04,00,20,00*09fd15d6\n\tsystem status\tnormal 2 28.000000 0 0\trobot status\t259.712506\t88.304900\t8.833600\t-0.400717\t-2.470513\t150.946486\t0.334000\t-0.046000\n\t\n15:35:05.6\tlog_raw\tgps_raw\t#INSPVAXA,USB3,0,50.0,FINESTEERING,2107,282923.600,02000000,471d,15824;INS_ALIGNMENT_COMPLETE,INS_RTKFIXED,37.37092659742,126.72376579558,8.8280,22.3000,0.2079,-0.2335,-0.0340,-0.348522367,-2.471236219,299.076821205,0.4391,0.2944,0.5534,0.1132,0.0924,0.0773,0.0980,0.1029,4.9102,0f000001,0*b1b4b9cc\n\tsystem status\tnormal 2 28.000000 0 0\trobot status\t259.595763\t88.384206\t8.828000\t-0.348522\t-2.471236\t150.923179\t0.335000\t-0.054000\n\t\n15:35:06.1\tlog_raw\tgps_raw\t#DUALANTENNAHEADINGA,USB3,0,50.0,FINESTEERING,2107,282924.100,02000000,d426,15824;INSUFFICIENT_OBS,NONE,-1.000000000,0.000000000,0.000000000,0.0,0.000000000,0.000000000,\"631T\",13,2,2,2,04,00,20,00*d3840d98\n\tsystem status\tnormal 2 28.000000 0 0\trobot status\t259.476998\t88.464105\t8.821800\t-0.401477\t-2.556277\t150.962011\t0.249000\t0.082000\n\t\n15:35:06.6\tlog_raw\tgps_raw\t#DUALANTENNAHEADINGA,USB3,0,51.0,FINESTEERING,2107,282924.600,02000000,d426,15824;INSUFFICIENT_OBS,NONE,-1.000000000,0.000000000,0.000000000,0.0,0.000000000,0.000000000,\"631T\",13,2,2,2,04,00,20,00*7b68c1aa\n\tsystem status\tnormal 2 28.000000 0 0\trobot status\t259.359956\t88.542489\t8.815500\t-0.491575\t-2.591134\t150.972893\t0.250000\t0.082000\n\t\n15:35:07.1\tlog_raw\tgps_raw\t#INSPVAXA,USB3,0,51.5,FINESTEERING,2107,282925.100,02008000,471d,15824;INS_ALIGNMENT_COMPLETE,INS_RTKFIXED,37.37092873619,126.72376179523,8.8090,22.3000,0.2069,-0.2351,-0.0215,-0.632285534,-2.693701140,299.016215129,0.4401,0.2945,0.5538,0.1133,0.0925,0.0773,0.0980,0.1029,4.9131,0f000001,0*70f1efa8\n\tsystem status\tnormal 2 28.000000 0 0\trobot status\t259.241418\t88.621588\t8.809000\t-0.632286\t-2.693701\t150.983785\t0.362000\t-0.083000\n\t\n15:35:07.6\tlog_raw\tgps_raw\t#DUALANTENNAHEADINGA,USB3,0,51.5,FINESTEERING,2107,282925.600,02008000,d426,15824;INSUFFICIENT_OBS,NONE,-1.000000000,0.000000000,0.000000000,0.0,0.000000000,0.000000000,\"631T\",13,2,2,2,04,00,20,00*5559a71e\n\tsystem status\tnormal 2 28.000000 0 0\trobot status\t259.124103\t88.700587\t8.803100\t-0.569231\t-2.829073\t150.996185\t0.311000\t-0.032000\n\t\n15:35:08.1\tlog_raw\tgps_raw\t#DUALANTENNAHEADINGA,USB3,0,49.5,FINESTEERING,2107,282926.100,02008000,d426,15824;INSUFFICIENT_OBS,NONE,-1.000000000,0.000000000,0.000000000,0.0,0.000000000,0.000000000,\"631T\",14,2,2,2,04,00,20,00*20bca12d\n\tsystem status\tnormal 2 28.000000 0 0\trobot status\t259.006675\t88.779598\t8.797200\t-0.565146\t-2.883992\t150.988138\t0.242000\t0.064000\n\t\n15:35:08.6\tlog_raw\tgps_raw\t#INSPVAXA,USB3,0,49.5,FINESTEERING,2107,282926.600,02008000,471d,15824;INS_ALIGNMENT_COMPLETE,INS_RTKFIXED,37.37093087426,126.72375780222,8.7912,22.3000,0.1944,-0.2057,-0.0172,-0.594741301,-2.946216927,299.056064983,0.4402,0.2946,0.5539,0.1133,0.0925,0.0773,0.0980,0.1029,4.9147,0f000001,0*64625386\n\tsystem status\tnormal 2 28.000000 0 0\trobot status\t258.887724\t88.858892\t8.791200\t-0.594741\t-2.946217\t150.943935\t0.348000\t-0.088000\n\t\n15:35:09.1\tlog_raw\tgps_raw\t#DUALANTENNAHEADINGA,USB3,0,49.5,FINESTEERING,2107,282927.100,02008000,d426,15824;INSUFFICIENT_OBS,NONE,-1.000000000,0.000000000,0.000000000,0.0,0.000000000,0.000000000,\"631T\",13,2,2,2,04,00,20,00*075a2ebf\n\tsystem status\tnormal 2 28.000000 0 0\trobot status\t258.770355\t88.938730\t8.785100\t-0.487639\t-2.949943\t150.882654\t0.290000\t0.002000\n\t\n15:35:09.6\tlog_raw\tgps_raw\t#INSPVAXA,USB3,0,51.0,FINESTEERING,2107,282927.600,02008000,471d,15824;INS_ALIGNMENT_COMPLETE,INS_RTKFIXED,37.37093229253,126.72375516206,8.7796,22.3000,0.1993,-0.2243,-0.0299,-0.537857110,-2.700770606,299.153411685,0.4404,0.2947,0.5542,0.1133,0.0925,0.0773,0.0980,0.1029,4.9162,0f000001,0*499bd090\n\tsystem status\tnormal 2 28.000000 0 0\trobot status\t258.653863\t89.016305\t8.779600\t-0.537857\t-2.700771\t150.846588\t0.295000\t0.002000\n\t\n15:35:10.1\tlog_raw\tgps_raw\t#DUALANTENNAHEADINGA,USB3,0,47.5,FINESTEERING,2107,282928.100,02008000,d426,15824;INSUFFICIENT_OBS,NONE,-1.000000000,0.000000000,0.000000000,0.0,0.000000000,0.000000000,\"631T\",16,2,2,2,04,00,20,00*2da4d93a\n\tsystem status\tnormal 2 28.000000 0 0\trobot status\t258.539041\t89.092914\t8.775300\t-0.654778\t-2.553226\t150.853471\t0.370000\t-0.104000\n\t\n15:35:10.6\tlog_raw\tgps_raw\t#DUALANTENNAHEADINGA,USB3,0,47.5,FINESTEERING,2107,282928.600,02008000,d426,15824;INSUFFICIENT_OBS,NONE,-1.000000000,0.000000000,0.000000000,0.0,0.000000000,0.000000000,\"631T\",16,2,2,2,04,00,20,00*e10cc3ac\n\tsystem status\tnormal 2 28.000000 0 0\trobot status\t258.423179\t89.169720\t8.772400\t-0.650140\t-2.305208\t150.878447\t0.260000\t0.066000\n\t\n15:35:11.1\tlog_raw\tgps_raw\t#INSPVAXA,USB3,0,50.5,FINESTEERING,2107,282929.100,02000000,471d,15824;INS_ALIGNMENT_COMPLETE,INS_RTKFIXED,37.37093438604,126.72375124490,8.7687,22.3000,0.1833,-0.2092,-0.0183,-0.594311335,-2.195857139,299.176557510,0.4400,0.2947,0.5540,0.1135,0.0926,0.0773,0.0980,0.1029,4.9192,0f000001,0*a006802b\n\tsystem status\tnormal 2 28.000000 0 0\trobot status\t258.306887\t89.248663\t8.768700\t-0.594311\t-2.195857\t150.823442\t0.282000\t0.017000\n\t\n15:35:11.6\tlog_raw\tgps_raw\t#INSPVAXA,USB3,0,50.5,FINESTEERING,2107,282929.600,02000000,471d,15824;INS_ALIGNMENT_COMPLETE,INS_RTKFIXED,37.37093510970,126.72374990284,8.7644,22.3000,0.1889,-0.2243,-0.0171,-0.596042414,-2.165494798,299.266591989,0.4400,0.2947,0.5540,0.1135,0.0926,0.0773,0.0980,0.1029,4.9192,0f000001,0*8915186d\n\tsystem status\tnormal 2 28.000000 0 0\trobot status\t258.188010\t89.328982\t8.764400\t-0.596042\t-2.165495\t150.733408\t0.283000\t0.022000\n\t\n15:35:12.1\tlog_raw\tgps_raw\t#INSPVAXA,USB3,0,50.5,FINESTEERING,2107,282930.100,02000000,471d,15824;INS_ALIGNMENT_COMPLETE,INS_RTKFIXED,37.37093581213,126.72374860624,8.7606,22.3000,0.1874,-0.2417,-0.0230,-0.681633205,-2.126475016,299.327076176,0.4420,0.2949,0.5548,0.1137,0.0926,0.0774,0.0980,0.1030,4.9200,0f000001,0*554adfff\n\tsystem status\tnormal 2 27.900000 0 0\trobot status\t258.073159\t89.406944\t8.760600\t-0.681633\t-2.126475\t150.672924\t0.300000\t0.009000\n\t\n15:35:12.6\tlog_raw\tgps_raw\t#INSPVAXA,USB3,0,50.5,FINESTEERING,2107,282930.600,02000000,471d,15824;INS_ALIGNMENT_COMPLETE,INS_RTKFIXED,37.37093652868,126.72374728704,8.7566,22.3000,0.1904,-0.2264,-0.0187,-0.696438502,-2.244688797,299.406875205,0.4420,0.2949,0.5548,0.1137,0.0926,0.0774,0.0980,0.1030,4.9200,0f000001,0*0f06850a\n\tsystem status\tnormal 2 28.000000 0 0\trobot status\t257.956307\t89.486474\t8.756600\t-0.696439\t-2.244689\t150.593125\t0.295000\t0.002000\n\t\n15:35:13.1\tlog_raw\tgps_raw\t#INSPVAXA,USB3,0,49.0,FINESTEERING,2107,282931.100,02000000,471d,15824;INS_ALIGNMENT_COMPLETE,INS_RTKFIXED,37.37093725237,126.72374594459,8.7526,22.3000,0.1776,-0.2170,-0.0174,-0.804539689,-2.256880287,299.491387164,0.4432,0.2951,0.5553,0.1137,0.0927,0.0774,0.0980,0.1030,4.9204,0f000001,0*08565520\n\tsystem status\tnormal 2 28.000000 0 0\trobot status\t257.837394\t89.566796\t8.752600\t-0.804540\t-2.256880\t150.508613\t0.255000\t0.062000\n\t\n15:35:13.6\tlog_raw\tgps_raw\t#DUALANTENNAHEADINGA,USB3,0,49.0,FINESTEERING,2107,282931.600,02000000,d426,15824;INSUFFICIENT_OBS,NONE,-1.000000000,0.000000000,0.000000000,0.0,0.000000000,0.000000000,\"631T\",13,2,2,2,04,00,20,00*c0d8f8a7\n\tsystem status\tnormal 2 28.000000 0 0\trobot status\t257.721167\t89.646576\t8.748400\t-0.860307\t-2.274262\t150.532811\t0.299000\t0.006000\n\t\n15:35:14.1\tlog_raw\tgps_raw\t#INSPVAXA,USB3,0,49.0,FINESTEERING,2107,282932.100,02000000,471d,15824;INS_ALIGNMENT_COMPLETE,INS_RTKFIXED,37.37093868529,126.72374334447,8.7450,22.3000,0.1876,-0.2264,-0.0189,-0.905927462,-2.146782726,299.477190532,0.4440,0.2953,0.5559,0.1139,0.0929,0.0774,0.0979,0.1030,4.9203,0f000001,0*aa1aa6b5\n\tsystem status\tnormal 2 28.000000 0 0\trobot status\t257.607080\t89.725835\t8.745000\t-0.905927\t-2.146783\t150.522809\t0.285000\t0.016000\n\t\n15:35:14.6\tlog_raw\tgps_raw\t#DUALANTENNAHEADINGA,USB3,0,51.0,FINESTEERING,2107,282932.600,02000000,d426,15824;INSUFFICIENT_OBS,NONE,-1.000000000,0.000000000,0.000000000,0.0,0.000000000,0.000000000,\"631T\",15,2,2,2,04,00,20,00*ae77645a\n\tsystem status\tnormal 2 28.000000 0 0\trobot status\t257.488163\t89.806345\t8.741500\t-0.877497\t-2.173506\t150.463190\t0.347000\t-0.091000\n\t\n15:35:15.1\tlog_raw\tgps_raw\t#DUALANTENNAHEADINGA,USB3,0,46.0,FINESTEERING,2107,282933.100,02000000,d426,15824;INSUFFICIENT_OBS,NONE,-1.000000000,0.000000000,0.000000000,0.0,0.000000000,0.000000000,\"631T\",15,2,2,2,04,00,20,00*38777e0f\n\tsystem status\tnormal 2 28.000000 0 0\trobot status\t257.371873\t89.887926\t8.737300\t-0.672611\t-2.219328\t150.456929\t0.310000\t-0.040000\n\t\n15:35:15.6\tlog_raw\tgps_raw\t#DUALANTENNAHEADINGA,USB3,0,46.0,FINESTEERING,2107,282933.600,02000000,d426,15824;INSUFFICIENT_OBS,NONE,-1.000000000,0.000000000,0.000000000,0.0,0.000000000,0.000000000,\"631T\",14,2,2,2,04,00,20,00*233de4c1\n\tsystem status\tnormal 2 28.000000 0 0\trobot status\t257.251774\t89.970275\t8.733300\t-0.715814\t-2.389524\t150.415727\t0.363000\t-0.098000\n\t\n15:35:16.1\tlog_raw\tgps_raw\t#DUALANTENNAHEADINGA,USB3,0,46.0,FINESTEERING,2107,282934.100,02000000,d426,15824;INSUFFICIENT_OBS,NONE,-1.000000000,0.000000000,0.000000000,0.0,0.000000000,0.000000000,\"631T\",15,2,2,2,04,00,20,00*e20e6641\n\tsystem status\tnormal 2 28.000000 0 0\trobot status\t257.135566\t90.052017\t8.728800\t-0.649437\t-2.351678\t150.405153\t0.252000\t0.074000\n\t\n15:35:16.6\tlog_raw\tgps_raw\t#DUALANTENNAHEADINGA,USB3,0,47.5,FINESTEERING,2107,282934.600,02000000,d426,15824;INSUFFICIENT_OBS,NONE,-1.000000000,0.000000000,0.000000000,0.0,0.000000000,0.000000000,\"631T\",17,2,2,2,04,00,20,00*6b2c4a4e\n\tsystem status\tnormal 2 28.000000 0 0\trobot status\t257.016499\t90.134498\t8.723700\t-0.746356\t-2.560496\t150.384460\t0.271000\t0.017000\n\t\n15:35:17.1\tlog_raw\tgps_raw\t#DUALANTENNAHEADINGA,USB3,0,47.5,FINESTEERING,2107,282935.100,02000000,d426,15824;INSUFFICIENT_OBS,NONE,-1.000000000,0.000000000,0.000000000,0.0,0.000000000,0.000000000,\"631T\",15,2,2,2,04,00,20,00*bee852f0\n\tsystem status\tnormal 2 28.000000 0 0\trobot status\t256.897483\t90.217013\t8.718700\t-0.854784\t-2.517054\t150.424391
